vi "Get_Notifier_Hault_Notifier.vi"(11 "Process Loop TypeDef (in)":T1 {"navX Device Memory Size" format="%x"; "Command Array" items=["UNDEFINED"=0, "NAVX_INTEGRATION_CTL_RESET_VEL_X"=1, "NAVX_INTEGRATION_CTL_RESET_VEL_Y"=2, "NAVX_INTEGRATION_CTL_RESET_VEL_Z"=4, "NAVX_INTEGRATION_CTL_RESET_DISP_X"=8, "NAVX_INTEGRATION_CTL_RESET_DISP_Y"=16, "NAVX_INTEGRATION_CTL_RESET_DISP_Z"=32, "NAVX_INTEGRATION_CTL_RESET_YAW"=128]; "I2CDevRef"."Device Address" format="%.0x"; "Device Info"."Interface"."Update Rate (4Hz-200Hz)" min=4 max=200 step=1}) -> (3 "Hault Notifier":bool)   [LabVIEW 2016]
uses:
  _TypeDefs/FRIC_navX_I2C Process Loop TypeDef.ctl
  _TypeDefs/FRIC_navX_ProcessingLoopStatesTypeDef_I2C.ctl
  _TypeDefs/Z900_navX_DeviceTypeDef.ctl
  _TypeDefs/Z900_navX_ProtocolTypeDef.ctl
  _TypeDefs/Z900_navX_NotifyPacketTypeDef.ctl
  _TypeDefs/Z900_navX_ActionTypeDef.ctl
  _TypeDefs/Z900_navX_SerialStreamTypeDef.ctl
  _TypeDefs/FRIC_navX_DeviceNumbersTypeDef.ctl
  <vilib>/Rock Robotics/SystemInterfaces/i2clib/i2c_bus.ctl
  _TypeDefs/Z900_navX_IntegrationControlRegisters.ctl
  <vilib>/Rock Robotics/WPI/SPI/WPI_SPIDevRef.ctl
  <vilib>/Rock Robotics/SystemInterfaces/spilib/spi_bus.ctl
  <vilib>/Rock Robotics/WPI/SerialPort/WPI_SerialPort.ctl
  <vilib>/Rock Robotics/WPI/SerialPort/WPI_SerialPortRef.ctl
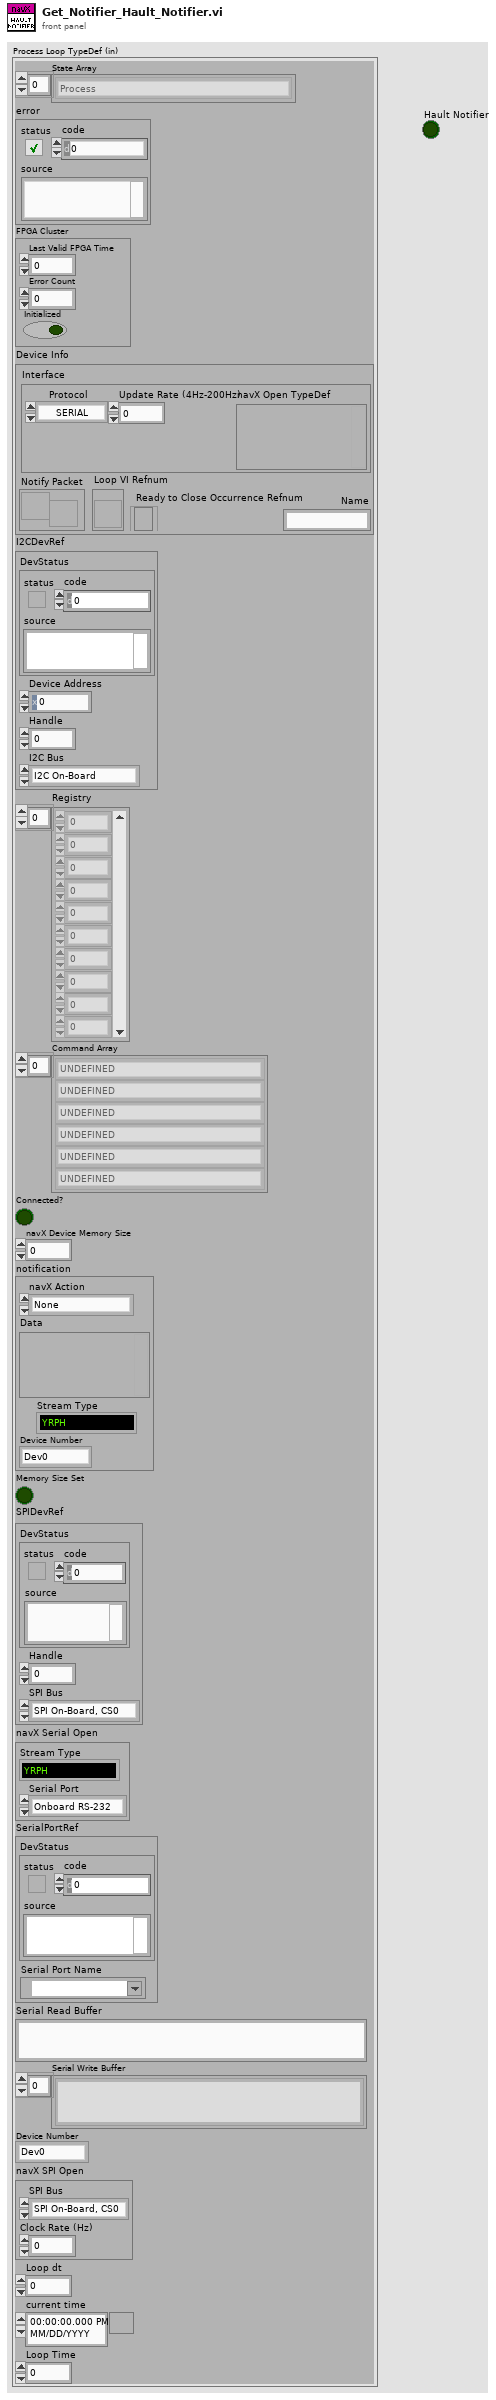
[diagram p1: front panel]
types:
  T1 = typedef "FRIC_navX_I2C Process Loop TypeDef.ctl" = cluster{"State Array":T2[], "error":errorcluster, "FPGA Cluster":cluster{"Last Valid FPGA Time":dbl, "Error Count":i32, "Initialized":bool}, "Device Info":T3, "I2CDevRef":cluster{"DevStatus":errorcluster, "Device Address":u8, "Handle":i32, "I2C Bus":T5}, "Registry":u8[], "Command Array":T6[], "Connected?":bool, "navX Device Memory Size":i32, "notification":T7, "Memory Size Set":bool, "SPIDevRef":T11, "navX Serial Open":cluster{"Stream Type":T9, "Serial Port":T13}, "SerialPortRef":T14, "Serial Read Buffer":string, "Serial Write Buffer":string[], "Device Number":T10, "navX SPI Open":cluster{"SPI Bus":T12, "Clock Rate (Hz)":dbl}, "Loop dt":i64, "current time":timestamp, "Loop Time":i64}
  T2 = typedef "FRIC_navX_ProcessingLoopStatesTypeDef_I2C.ctl" = enum16{"Process", "INI", "Check Packets Valid", "Close", "Flush Serial", "Generate Command", "Last Packet Valid", "Open", "Read", "Reset Serial", "Set Termination Char", "Update AE", "Wait", "Write", "Exit"}
  T3 = typedef "Z900_navX_DeviceTypeDef.ctl" = cluster{"Interface":cluster{"Protocol":T4, "Update Rate (4Hz-200Hz)":u8, "navX Open TypeDef":variant}, "Notify Packet":refnum<notifier>, "Loop VI Refnum":refnum<vi>, "Ready to Close Occurrence Refnum":refnum<k4>, "Name":string}
  T4 = typedef "Z900_navX_ProtocolTypeDef.ctl" = enum16{"SERIAL", "I2C", "SPI"}
  T5 = typedef "i2c_bus.ctl" = enum16{"I2C On-Board", "I2C MXP", "Invalid"}
  T6 = typedef "Z900_navX_IntegrationControlRegisters.ctl" = u8
  T7 = typedef "Z900_navX_NotifyPacketTypeDef.ctl" = cluster{"navX Action":T8, "Data":variant, "Stream Type":T9, "Device Number":T10}
  T8 = typedef "Z900_navX_ActionTypeDef.ctl" = enum16{"None", "Halt", "Normal Read", "Update Serial Protocol", "Update Rate Htz", "Zero-Yaw", "Zero-Displacement", "Zero-Velocity"}
  T9 = typedef "Z900_navX_SerialStreamTypeDef.ctl" = enum16{"YRPH", "Quaterinons", "Gyro/Raw", "AHRS", "AHRSAndPositioning", "AHRSAndPOSTime"}
  T10 = typedef "FRIC_navX_DeviceNumbersTypeDef.ctl" = enum16{"Dev0", "Dev1", "Dev2", "Dev3", "Dev4", "Dev5", "Dev6", "Dev7", "Dev8", "Dev9", "Dev10"}
  T11 = typedef "WPI_SPIDevRef.ctl" = cluster{"DevStatus":errorcluster, "Handle":i32, "SPI Bus":T12}
  T12 = typedef "spi_bus.ctl" = enum16{"SPI On-Board, CS0", "SPI On-Board, CS1", "SPI On-Board, CS2", "SPI On-Board, CS3", "SPI MXP", "Invalid"}
  T13 = typedef "WPI_SerialPort.ctl" = enum16{"Onboard RS-232", "MXP TTL", "USB 1", "USB 2"}
  T14 = typedef "WPI_SerialPortRef.ctl" = cluster{"DevStatus":errorcluster, "Serial Port Name":refnum<visa-resource-name>}
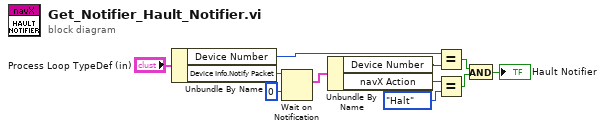
[diagram p0: block diagram]
diagram:
  n1 = Unbundle By Name("Process Loop TypeDef (in)") -> ("Device Number"=w10:T10, "Device Info.Notify Packet"=w6:refnum<notifier>)
  n2 = Wait on Notification(notifier=w6, timeout in ms (-1)=0) -> (notification=w9:T7)  [unwired: 2 in, 3 out]
  n3 = Unbundle By Name(w9) -> ("Device Number"=w11:T10, "navX Action"=w5:T8)
  n4 = Equal?(x=w10, y=w11) -> (x = y?=w2:bool)
  n5 = Equal?(x=w5, y=Z900_navX_ActionTypeDef."Halt") -> (x = y?=w1:bool)
  n6 = And(x=w2, y=w1) -> (x .and. y?=→"Hault Notifier":bool)
